vi "CLSUIP_MakeTermsMatchIconState.vi"(8 "error in (no error)":errorcluster, 10 "Terminal":refnum<vi>, 11 "VI Refnum":refnum<vi>) -> (0 "error out":errorcluster, 3 "VI Refnum out":refnum<vi>)   [LabVIEW 2021, in "MemberVICreation.lvlib"]
uses:
  <resource>/Framework/Providers/LVClassLibrary/NewAccessors/MemberVICreation.lvlib
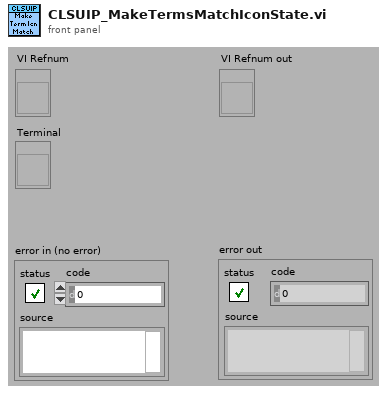
[diagram p1: front panel]
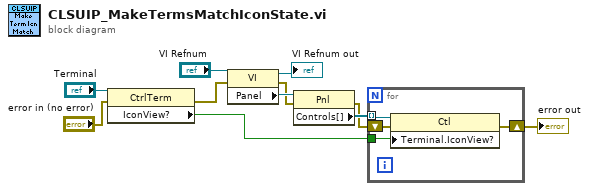
[diagram p0: block diagram]
diagram:
  n1 = property class="CtrlTerm"(reference="Terminal", error in="error in (no error)") -> (error out=w5:errorcluster, "IconView?"=w1:bool)  [unwired: 1 out]
  n2 = property class="VI"(reference="VI Refnum", error in=w5) -> (reference out=→"VI Refnum out":refnum<vi>, error out=w6:errorcluster, "Panel"=w9:refnum<vi>)
  n3 = property class="Pnl"(reference=w9, error in=w6) -> (error out=w3:errorcluster, "Controls[]"=w4:refnum<vi>[])  [unwired: 1 out]
  n4 = for {
    tunnel: w4 -> [w14] mode=indexing
    shift-right: [w13] -> w2
    shift-left: w3 -> [w15]
    tunnel: w1 -> [w12]
    n5 = property class="Ctl"(reference=w14, error in=w15, "Terminal.IconView?"=w12) -> (error out=w13:errorcluster)  [unwired: 1 out]
  }
  "error out" <- w2
